vi "Práctica8_Procesos.vi"() -> ()   [LabVIEW 2018]
panel:
  out "Ejecución":dbl
  out "Presentación":u8(slide) scale=0.0..100.0
  out "Etapa 2":bool
  out "Etapa1":bool
  in  "Pedido":dbl
  in  "stop":bool
  out "Fórmula\nsecreta":dbl(slide) scale=0.0..2600.0
  out "Hielo":dbl(slide) scale=0.0..5000.0
  out "Agua \npurificada":dbl(slide) scale=0.0..10000.0
  out "Saborizante \ncolorante":dbl(slide) scale=0.0..1300.0
  # "Anahí Montserrat Vázquez Padilla\nMiércoles 20 de marzo del 2024 \nPráctica 9. Diseño"
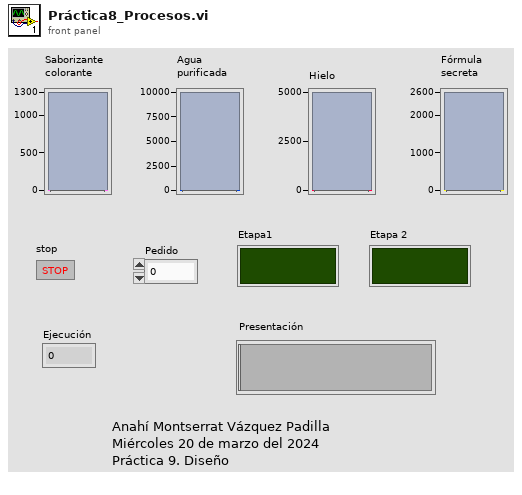
[diagram p1: front panel]
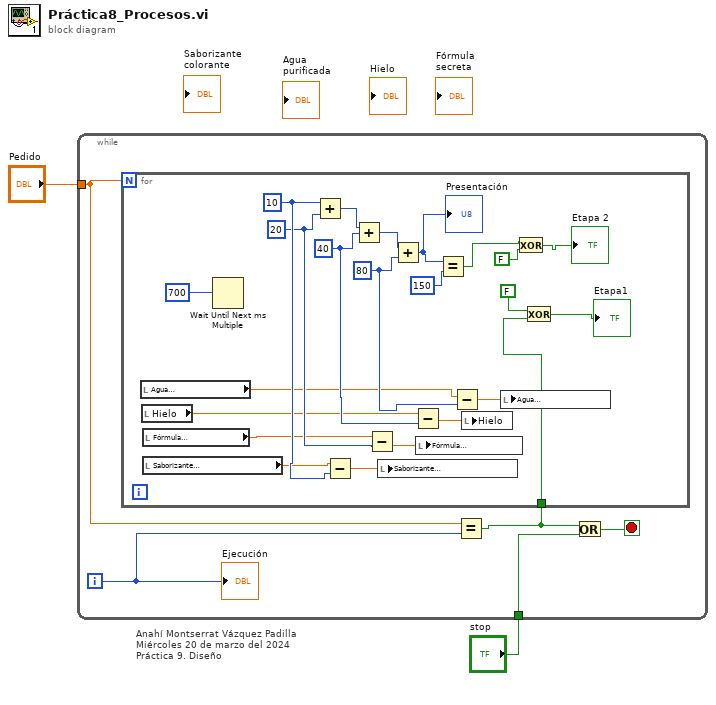
[diagram p0: block diagram]
diagram:
  # "Anahí Montserrat Vázquez Padilla\nMiércoles 20 de marzo del 2024 \nPráctica 9. Diseño"
  n1 = while {
    tunnel: "Pedido" -> [w7]
    tunnel: "stop" -> [w5]
    i -> [w3]
    stop <- w6 stop-if-true
    n2 = Equal?(x=w7, y=w3) -> (x = y?=w4:bool)
    n3 = for {
      N: w7 -> [_]
      tunnel: w4 -> [w17]
      w10 = 80
      w12 = 40
      w14 = 20
      w16 = 10
      n4 = local read "Agua \npurificada"() -> (w9:dbl)
      n5 = local read "Hielo"() -> (w11:dbl)
      n6 = local read "Fórmula\nsecreta"() -> (w13:dbl)
      n7 = local read "Saborizante \ncolorante"() -> (w15:dbl)
      n8 = Wait Until Next ms Multiple(millisecond multiple=700) -> ()  [unwired: 1 out]
      n9 = Add(x=w16, y=w14) -> (x+y=w30:i32)
      n10 = Subtract(x=w15, y=w16) -> (x-y=w28:dbl)
      n11 = Add(x=w30, y=w12) -> (x+y=w29:i32)
      n12 = Subtract(x=w13, y=w14) -> (x-y=w27:dbl)
      n13 = local write "Saborizante \ncolorante"(w28) -> ()
      n14 = Add(x=w29, y=w10) -> (x+y=w24:i32)
      "Presentación" <- w24
      n15 = Subtract(x=w11, y=w12) -> (x-y=w26:dbl)
      n16 = local write "Fórmula\nsecreta"(w27) -> ()
      n17 = Equal?(x=w24, y=150) -> (x = y?=w21:bool)
      n18 = Subtract(x=w9, y=w10) -> (x-y=w25:dbl)
      n19 = local write "Hielo"(w26) -> ()
      n20 = local write "Agua \npurificada"(w25) -> ()
      n21 = Exclusive Or(1:FALSE, 2:w21) -> (0:→"Etapa 2":bool)
      n22 = Exclusive Or(1:w17, 2:FALSE) -> (0:→"Etapa1":bool)
    }
    n23 = Or(x=w4, y=w5) -> (x .or. y?=w6:bool)
    "Ejecución" <- w3
  }
